vi "determineIfUseWeakForce.vi"(6 "pass?":bool=TRUE, 8 "error in (no error)":errorcluster, 9 "EnableWeakKick":bool, 10 "Game":refnum<class "Game.lvclass">, 11 "KickToSkill in":refnum<class "KickToSkill.lvclass">) -> (0 "error out":errorcluster, 2 "canWeakKick":bool, 3 "KickToSkill out":refnum<class "KickToSkill.lvclass">)   [LabVIEW 2023, in "KickToSkill.lvclass"]
uses:
  KickToSkill.lvclass
  Game_class/Game.lvclass
  Robot_class/Robot.lvclass
  C:/Users/lucio/Desktop/roboime/SSL_AI/Object_class/Object.lvclass
  Team_class/OffensivePlay.ctl
  Game_class/Game.lvclass/Game.ctl
  Parameters_class/Parameters.lvclass/Parameters.ctl
  Team_class/Team.lvclass/Team.ctl
  Object_class/Object.lvclass/Object.ctl
  Object_class/Read x.vi
  Object_class/Read position(x,y).vi
  Game_class/Read BallRef.vi
  Game_class/Read Parameters.lvclass.vi
  Game_class/Read NewParameters.vi
  Game_class/Read FieldRef.vi
  Game_class/Read EnemyRef.vi
  Game_class/Read OffensiveTeam.vi
  Team_class/Read OffensivePlay.vi
  Team_class/Read RobotRef.vi
  Parameters_class/Read AttakingOurselves.vi
  Ally_class/Ally.lvclass
  C:/Users/lucio/Desktop/roboime/SSL_AI/Team_class/Team.lvclass
  Enemy_class/Enemy.lvclass
  Ball_class/Ball.lvclass
  Parameters_class/Parameters.lvclass
  Field_class/Field.lvclass
  Utilities_class/Utilities.lvclass
panel:
  in  "Robot":refnum<class "Robot.lvclass">
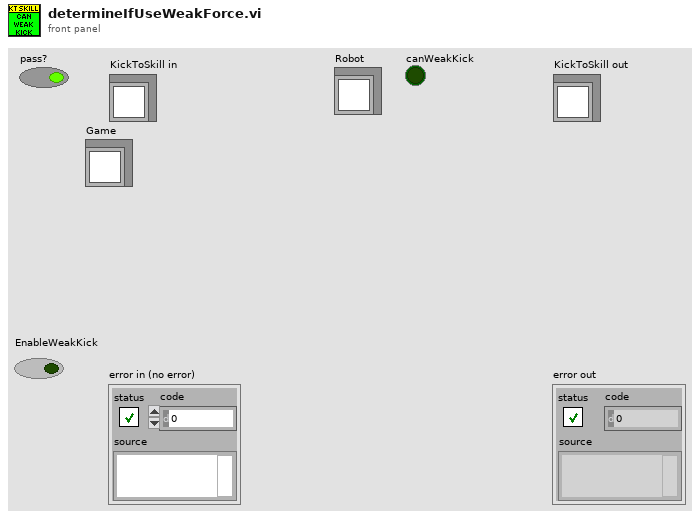
[diagram p1: front panel]
types:
  T1 = typedef "OffensivePlay.ctl" = enum16{"5RobotsPassGamePlay", "5PreparePassGame", "5RobotsKeeperGame", "KeeperPassToStriker", "5RobotsNormalGamePlay", "PrepareKeeperPass", "ACBPass", "ABCPass", "PrepareTriplePass", "TableWithStriker", "TableWith2ndStrikerPlay", "PrepareDoublePass", "PrepareRollToPass", "SimplePass", "PreparePass", "PassToStriker", "BallOutOfField", "PassTo2ndStriker", "StopOffensive", "Prepare Penalty Enemy", "EnemyPossessionAtEnemyField", "EnemyPossesionAtOurField", "TestPlay", "PreparePenaltyAlly", "KickPenaltyAlly", "PrepareKickoffAlly", "PrepareKickoffEnemy", "IndirectEnemy", "DirectEnemy", "PreparePassInGame1", "NormalGame", "DirectKick", "Pass", "Halt", "Timeout", "PassPlay", "PenaltyEnemy"}
  T2 = typedef "NewParameters.ctl" = cluster{"PenaltyDistance":dbl, "DistanceAttackerToBackBall":dbl, "Division":enum16{"Div B", "Div A"}, "DistanceToAvoidyEnemyRobot":dbl, "BallPlacementDistance":dbl, "DisatanceBehindBallToStealBall":dbl, "MaxDistanceToPositionKickoff":dbl, "BlockEnemyTarget":bool, "MaxStopVAng":dbl, "DistanceMarkerToEnemy":dbl, "IgnoreDribblerContact":bool, "DistanceToBeginEnemyPosession":dbl, "GoToBallWhenEnemyNotMoving":bool, "EnemyDistanceToReduceVelocity":dbl, "TurnOnEnemyDistanceToReduceVelocity":bool, "EnemyDistanceToShootOutBall":dbl, "DefenseKickBall":bool, "MoreKickToGoal? (0-0.3)":dbl, "ChipKickInEnemyField":bool, "ShootOutRobotId":dbl, "FieldLenghtDenominatorInShootOut":dbl, "AdjustPositionInBallPlacement":bool, "PowerGodPass":dbl, "VelocityAbortEnemyPos":dbl, "MaxDistToBeginPass":dbl, "MinDistToBeginPass":dbl, "VelocityInDirects":dbl, "BadDribblerIDs":i32[], "NewKickToDistanceAroundBall":dbl, "PowerAvoidColisionMarker":dbl, "DistanceToAvoidColisionMarker":dbl, "AvoidBallKick":dbl, "DistanceTryKick":dbl, "SuicideKickDIstance":dbl, "AdjustFirstKickDistance":dbl, "AvoidAimLessKick":dbl, "DistanceToAvoidyEnemyShootRobot ":dbl, "NumberOfMarkers":dbl, "PotField":bool, "PIDLateral":bool, "MinDistanceFirstKickX":dbl, "MinDistanceFirstKickY":dbl, "FractionOfDistToTouchGround\nAfterChipKick":dbl, "FractionOfKickxWhen\nComposedWithKickz":dbl, "Style":T3, "MoveInTurnState":bool, "DistFromEnemyToConsider\nMoveInTurnState":dbl, "CascadePID":bool, "TurnAroundParameters":cluster{"Radius":dbl, "Multiplier":dbl, "ChordAngle":dbl}, "SafeDriveVel":dbl, "DistanceToGoToBackBall":dbl, "minDistanceToNotFinish\nEnemyPossession":dbl, "OneTouchShot":cluster{"angleFactor":dbl, "maxAngle":dbl, "Attack":bool, "Defense":bool}, "OpenAngleToGoal":cluster{"minAngle":dbl, "maxAngle":dbl, "minEvaluation":dbl}, "ShotInterception":cluster{"shotSpeed":dbl, "minEnemySpeed":dbl, "maxEnemySpeed":dbl, "minEvaluation":dbl}, "AllyTeamArray":T4[], "maxDefendersNumber":i32, "Zone":cluster{"GuardPositionArray":dbl[][], "ZoneMidField":dbl[], "CenterForwardWidth":dbl}, "MinEvaluationToShoot":dbl, "PassInterception":cluster{"maxPassSpeed":dbl, "minPassSpeed":dbl, "minEnemySpeed":dbl, "chipPassDistance":dbl, "chipPassEvaluation":dbl, "minEvaluation":dbl, "maxEnemySpeed":dbl}, "PassDistance":cluster{"maxDistance":dbl, "minDistance":dbl}, "receiverSpeed":dbl, "maxBallSpeed":dbl, "slackTime":dbl, "Turning radius":dbl, "Turning v_ang":dbl, "AlignError":cluster{"Distance":dbl, "Orientation":dbl, "V_norm(m/s)":dbl, "V_ang (rad/s)":dbl}, "RobotRadius":dbl, "KickerDistance":dbl, "keeper angle  to cover goalpost":dbl}
  T3 = typedef "Style.ctl" = enum16{"Insanity", "Offensive", "Defensive"}
  T4 = typedef "AllyTeam.ctl" = enum16{"Keeper", "Defender", "Attacker"}
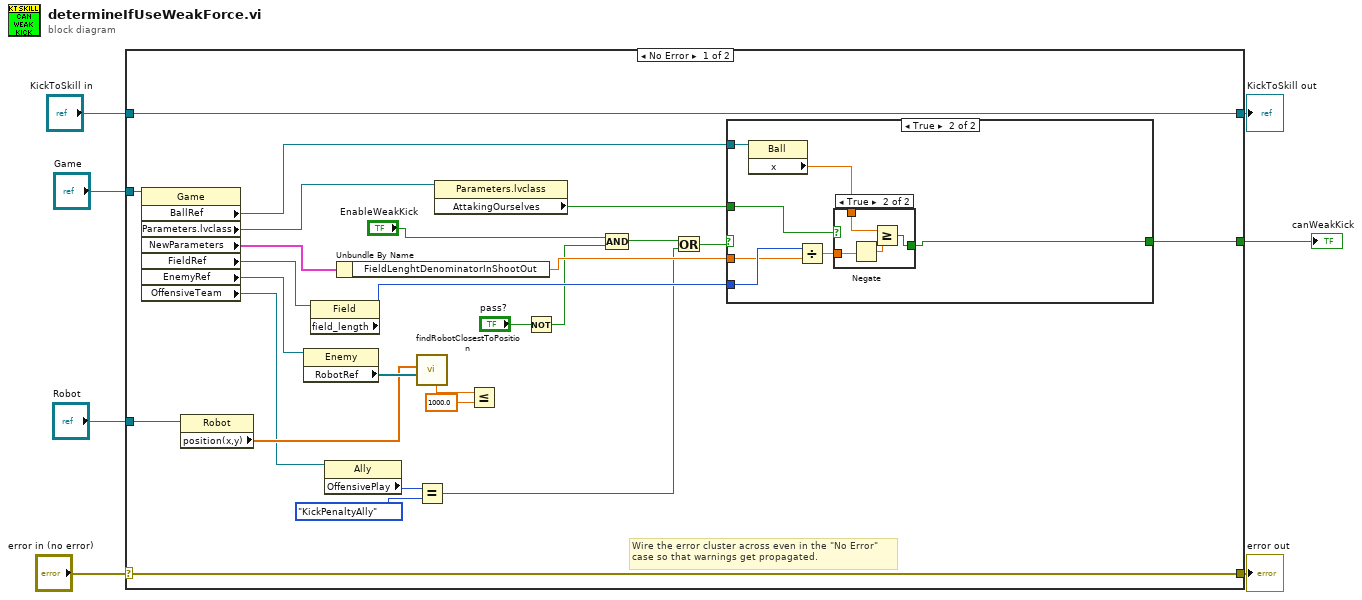
[diagram p0: block diagram]
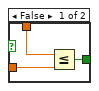
[diagram p3: hidden frame]
diagram:
  n1 = case shown="No Error" "error in (no error)" {
    selector: "error in (no error)" -> [w32 w50]
    tunnel: [w32 w50] -> w6
    tunnel: [w33 w49] -> w4
    tunnel: "KickToSkill in" -> [w33 w49]
    tunnel: "Game" -> [w28 _]
    tunnel: [w23 _] -> w2
    tunnel: "Robot" -> [w17 _]
    frame No Error {
      # "Wire the error cluster across even in the \"No Error\"\ncase so that warnings get propagated."
      n2 = property class="Game"(reference=w28) -> ("BallRef"=w27:refnum<class "Ball.lvclass">, "Parameters.lvclass"=w26:refnum<class "Parameters.lvclass">, "NewParameters"=w25:T2, "FieldRef"=w24:refnum<class "Field.lvclass">, "EnemyRef"=w19:refnum<class "Enemy.lvclass">, "OffensiveTeam"=w11:refnum<class "Ally.lvclass">)  [unwired: 1 in, 2 out]
      n3 = property class="Robot"(reference=w17) -> ("position(x,y)"=w16:dbl[])  [unwired: 1 in, 2 out]
      n4 = property class="Enemy"(reference=w19) -> ("RobotRef"=w18:refnum<class "Robot.lvclass">[])  [unwired: 1 in, 2 out]
      n5 = property class="Field"(reference=w24) -> ("field_length"=w29:i32)  [unwired: 1 in, 2 out]
      n6 = property class="Ally"(reference=w11) -> ("OffensivePlay"=w10:T1)  [unwired: 1 in, 2 out]
      n7 = Unbundle By Name(w25) -> ("FieldLenghtDenominatorInShootOut"=w30:dbl)
      n8 = call "findRobotClosestToPosition.vi"("robotsArray"=w18, "position"=w16) -> ("Distance"=w15:dbl)  [unwired: 5 in, 4 out]
      n9 = Equal?(x=w10, y=OffensivePlay."KickPenaltyAlly") -> (x = y?=w8:bool)
      n10 = property class="Parameters.lvclass"(reference=w26) -> ("AttakingOurselves"=w31:bool)  [unwired: 1 in, 2 out]
      n11 = Less Or Equal?(x=w15, y=1000.0) -> ()  [unwired: 1 out]
      n12 = Not(x="pass?") -> (.not. x?=w20:bool)
      n13 = Compound Arithmetic op=AND("EnableWeakKick", w20) -> (w12:bool)
      n14 = Or(x=w12, y=w8) -> (x .or. y?=w13:bool)
      n15 = case shown="True" w13 {
        selector: w13 -> [w34 _]
        tunnel: w29 -> [_ w41]
        tunnel: w27 -> [_ w39]
        tunnel: w31 -> [_ w37]
        tunnel: w30 -> [_ w36]
        tunnel: [w34 w35] -> w23
        frame False {
        }
        frame True {
          n16 = property class="Ball"(reference=w39) -> ("x"=w38:dbl)  [unwired: 1 in, 2 out]
          n17 = Divide(x=w41, y=w36) -> (x/y=w40:dbl)
          n18 = case shown="True" w37 {
            tunnel: w40 -> [w44 w48]
            tunnel: w38 -> [w43 w45]
            tunnel: [w42 w47] -> w35
            frame False {
              n19 = Less Or Equal?(x=w43, y=w44) -> (x <= y?=w42:bool)
            }
            frame True {
              n20 = Negate(x=w48) -> (-x=w46:dbl)
              n21 = Greater Or Equal?(x=w45, y=w46) -> (x >= y?=w47:bool)
            }
          }
        }
      }
    }
    frame Error {
    }
  }
  "error out" <- w6
  "KickToSkill out" <- w4
  "canWeakKick" <- w2
